vi "Database Insert.vi"() -> ()   [LabVIEW 2013]
doc: "This example allows you to perform several tasks on the specified table in a database named LabVIEW.mdb located in the LabVIEW examples>>database directory.\n\nThis VI is running when you open it. Select one of the tabs and enter the appropriate data. Press the Go button to complete the displayed tab option.\n\nAutomatic - This option inserts a new record into the specified table. The record is specified by a cluster containing the correct number of elements and of the data types defined by the specified table. \n\nSQL Query - This option performs the specified SQL query.\n\nParameterized SQL Query - This option performs the specified SQL query as a parameterized SQL Query. This method is faster and more efficient than directly executing an SQL query because it sets up all the parameters prior to doing the command."
uses:
  Auxilliary.llb/DB Tools Parameter Info.ctl
  Auxilliary.llb/DB Tools DataTypes.ctl
  Auxilliary.llb/DB Tools Parameter Dir.ctl
  Connection.llb/DB Tools Open Connec (Path).vi
  Connection.llb/Conn Execute.vi
  Recordset.llb/Rec Destroy - Connection.vi
  Command.llb/Cmd Set Parameter Value (C).vi
  Command.llb/Cmd Execute.vi
  Recordset.llb/Rec Destroy - Command.vi
  Command.llb/Cmd Delete.vi
  NI_Database_API_64.lvlib
panel:
  in  "GO Button":bool
  in  "Table":string="inserttable"
  in  "Tab Control":T1(tab)=enum."Parameterized SQL Query"
  in  "Data":T2={"query type"="automatic", "device name"="mydevice", "number of samples"=1024}
  in  "SQL query":string="insert into inserttable (querytype, device, numsamples) values ('sql query', 'mydevice', 1872) "
  in  "number of samples":i32=2048
  in  "device name":string="mydevice"
  in  "parameters":T3[](array[typedef])=[{"parameter name"="", "type"=enum."String", "direction"=enum."Input", "value"=variant}, {"parameter name"="", "type"=enum."Long (I32)", "direction"=enum."Input", "value"=variant}]
  in  "parameterized SQL query":string="insert into inserttable (querytype, device, numsamples) values ('parameterized sql query', ?, ?) "
  # "INSTRUCTIONS:\n\nChoose which method to use to insert data into the table by clicking the corresponding tab.\n\nHit the GO button to execute.  You do not have to change any of the data in the controls as they are already set up correctly."
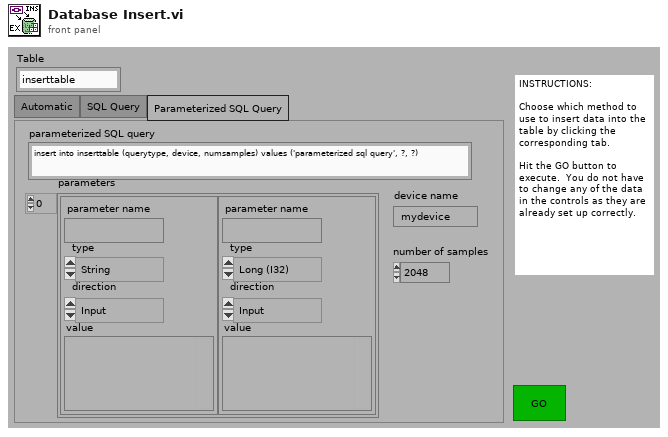
[diagram p1: front panel]
types:
  T1 = enum32{"Automatic", "SQL Query", "Parameterized SQL Query"}
  T2 = cluster{"query type":string, "device name":string, "number of samples":i32}
  T3 = typedef "NI_Database_API_64.lvlib/DB Tools Parameter Info.ctl" = cluster{"parameter name":string, "type":T4, "direction":T5, "value":variant}
  T4 = typedef "NI_Database_API_64.lvlib/DB Tools DataTypes.ctl" = enum16{"String", "Long (I32)", "Single (SGL)", "Double (DBL)", "Date/Time", "Binary"}
  T5 = typedef "NI_Database_API_64.lvlib/DB Tools Parameter Dir.ctl" = enum32{"Input", "Output", "Input/Output", "Return Value"}
  T6 = typedef "NI_Database_API_64.lvlib/Conn ObjectReference.ctl" = refnum<k1>
  T7 = typedef "NI_Database_API_64.lvlib/Rec ObjectReference.ctl" = refnum<k1>
  T8 = typedef "NI_Database_API_64.lvlib/Cmd ObjectReference.ctl" = refnum<k1>
  T9 = typedef "NI_Database_API_64.lvlib/Cmd-Rec Object Reference.ctl" = refnum<k1>
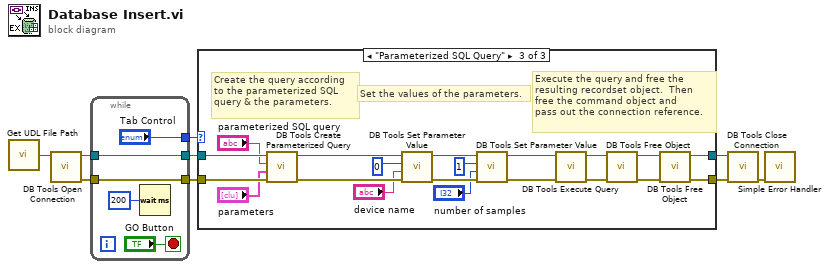
[diagram p0: block diagram]
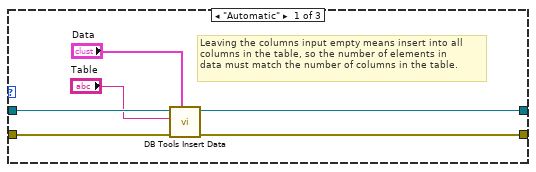
[diagram p2: hidden frame]
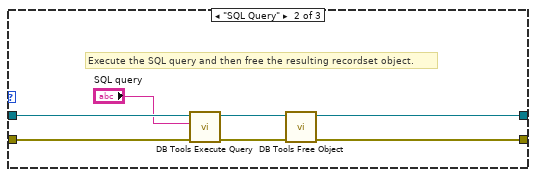
[diagram p3: hidden frame]
diagram:
  n1 = call "Get UDL File Path.vi"() -> ("UDL file path"=w2:path)  [unwired: 1 in]
  n2 = call-poly "DB Tools Open Connection.vi"("connection information"=w2) -> ("error out"=w5:errorcluster, "connection reference"=w6:T6)  [unwired: 7 in]
  n3 = while {
    tunnel: ["Tab Control"] -> w9
    tunnel: [w12] -> w7
    tunnel: w6 -> [w12]
    tunnel: w5 -> [w11]
    tunnel: [w11] -> w4
    stop <- "GO Button" stop-if-true
    n4 = Wait (ms)(milliseconds to wait=u32 200) -> ()  [unwired: 1 out]
  }
  n5 = case shown="\"Parameterized SQL Query\"" w9 {
    tunnel: w4 -> [w20 w23 w45]
    tunnel: w7 -> [w19 w24 w46]
    tunnel: [w18 w25 w44] -> w8
    tunnel: [w15 w21 w28] -> w1
    frame "Automatic" {
      # "Leaving the columns input empty means insert into all\ncolumns in the table, so the number of elements in\ndata must match the number of columns in the table."
      n6 = call "DB Tools Insert Data.vi"("data"="Data", "error in (no error)"=w20, "table"="Table", "connection reference"=w19) -> ("error out"=w18:errorcluster, "connection reference out"=w15:T6)  [unwired: 6 in]
    }
    frame "SQL Query" {
      # "Execute the SQL query and then free the resulting recordset object."
      n7 = call-poly "DB Tools Execute Query.vi"("error in (no error)"=w23, "SQL query"="SQL query", "connection reference"=w24) -> ("error out"=w27:errorcluster, "recordset reference"=w26:T7)  [unwired: 5 in]
      n8 = call-poly "DB Tools Free Object.vi"("error in (no error)"=w27, "recordset reference"=w26) -> ("error out"=w25:errorcluster, "connection reference"=w21:T6)  [unwired: 8 in]
    }
    frame "Parameterized SQL Query" {
      # "Execute the query and free the \nresulting recordset object.  Then \nfree the command object and \npass out the connection reference."
      # "Set the values of the parameters."
      # "Create the query according \nto the parameterized SQL \nquery & the parameters."
      n9 = call "DB Tools Create Parameterized Query.vi"("error in (no error)"=w45, "parameters"="parameters", "SQL query"="parameterized SQL query", "connection reference"=w46) -> ("error out"=w42:errorcluster, "command reference"=w34:T8)  [unwired: 3 in, 1 out]
      n10 = call-poly "DB Tools Set Parameter Value.vi"("error in (no error)"=w42, "value"="device name", "parameter index"=0, "command reference"=w34) -> ("error out"=w40:errorcluster, "command reference out"=w41:T8)  [unwired: 4 in]
      n11 = call-poly "DB Tools Set Parameter Value.vi"("error in (no error)"=w40, "value"="number of samples", "parameter index"=1, "command reference"=w41) -> ("error out"=w31:errorcluster, "command reference out"=w32:T8)  [unwired: 4 in]
      n12 = call-poly "DB Tools Execute Query.vi"("error in (no error)"=w31, "command reference"=w32) -> ("error out"=w33:errorcluster, "command-recordset reference"=w30:T9)  [unwired: 6 in]
      n13 = call-poly "DB Tools Free Object.vi"("error in (no error)"=w33, "command-recordset reference"=w30) -> ("error out"=w44:errorcluster, "command reference"=w29:T8)  [unwired: 8 in]
      n14 = call-poly "DB Tools Free Object.vi"("error in (no error)"=w44, "command reference"=w29) -> ("connection reference"=w28:T6)  [unwired: 8 in, 1 out]
    }
  }
  n15 = call "DB Tools Close Connection.vi"("error in (no error)"=w8, "connection reference"=w1) -> ("error out"=w3:errorcluster)  [unwired: 5 in]
  n16 = call <vilib>:"Simple Error Handler.vi"("error in (no error)"=w3) -> ()  [unwired: 4 in, 5 out]
